vi "Revision Query.vi"(8 "error in (no error)":errorcluster, 11 "Maxon Encoder in":refnum<class "Maxon Encoder.lvclass">) -> (0 "error out":errorcluster, 2 "Sensor Driver Revision":string, 3 "Maxon Encoder out":refnum<class "Maxon Encoder.lvclass">)   [LabVIEW 2019, in "Maxon Encoder.lvclass"]
doc: "Queries the current sensor driver revision.\n\nRefer to the Readme file for detailed driver information including modification history."
uses:
  Maxon Encoder.lvclass
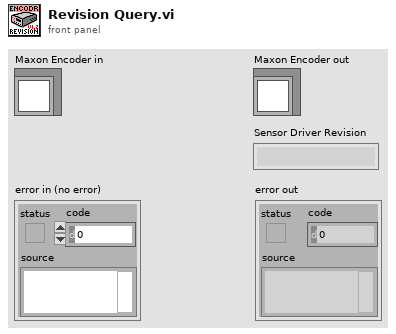
[diagram p1: front panel]
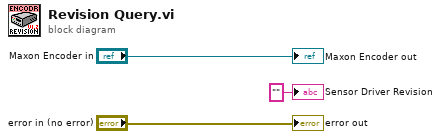
[diagram p0: block diagram]
diagram:
  "Sensor Driver Revision" <- "" ("Sensor Driver Revision")
  "error out" <- "error in (no error)"
  "Maxon Encoder out" <- "Maxon Encoder in"
